vi "Main_v4.vi"() -> ()   [LabVIEW 2016]
uses:
  <vilib>/Analysis/Matrix/Datatypes/RealMatrix.ctl
  subVIs/Global Variables.vi
  <vilib>/picture/3D Picture Control/Helpers/Apply Texture (no reference).vi
  <vilib>/picture/3D Picture Control/NI_3D Picture Control.lvlib
  <vilib>/Analysis/Matrix/NI_Matrix.lvlib
panel:
  in  "Run 2":bool=TRUE
  in  "Refresh Button":bool
  out "Ready?":bool
  in  "Done":bool
  in  "Help":bool
  in  "Abort":bool
  in  "Run":bool
  out "Estimated Time\nfor Lithography":timestamp=timestamp(-68372.87678205769 s since 1904-01-01) format="%<%H:%M:%S>T"
  in  "Visualization":T1(tab)
  out "Render":T2(plugin-control)
  out "Voltage Mapping":dbl(ramp)
  out "2D":T2(plugin-control)
  out "3D Picture":refnum<vi>(3d-picture)
  in  "Settings":T3(tab)
  in  "interpolation distance":dbl=0.1
  in  "Lithography Config File (.lcf)":path=path "P:/users1/Akash/Old/Akash AFM/Test Images/Sample AFM SVGs/2 electrode Writing Test.svg"
  in  "Patterns (drag-and-drop reorder)":i32(listbox)
  in  "image data max":dbl(slide)=100.0 min=0.0 max=100.0 scale=0.0..100.0
  in  "image data min":dbl(slide)=17.365269461077844 min=0.0 max=100.0 scale=0.0..100.0
  in  "AFM Type":u16(ring)=1 items=["Cypher", "MFP3D", "MFP3D_Lucy", "Simulation"]
  in  "Page":i32=1 min=0
  in  "Inkscape File (.svg)":path=path "\\\\synology.phyast.pitt.edu\\public/users1/Yuhe/cypher/1D Coulomb Drag_single QPC.svg"
  in  "Background Image":path=path "\\\\synology.phyast.pitt.edu\\public/users1/Yuhe/AFM scanned images/20170708/SA2821D0001.ibw"
  # "``"
  # "Before you start the program\nchange these paths to the\ncorresponding files"
  # "In simulation mode, to change the perspective, hold the left button of mouse and drag in the picture.\nTo zoom in and out, hold the shift button, hold the left button of the mouse and drag up and down in\nthe picture."
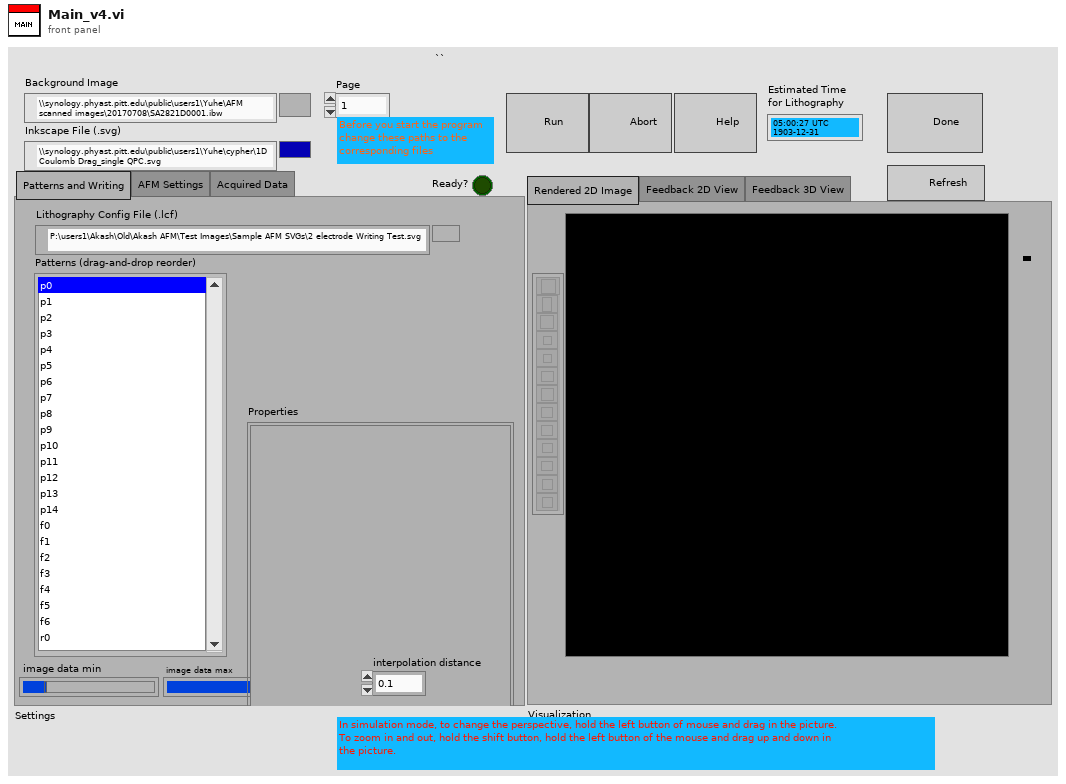
[diagram p1: front panel]
types:
  T1 = enum32{"Rendered 2D Image", "Feedback 2D View", "Feedback 3D View"}
  T2 = typedef "IMAQ Image.ctl" = refnum<image>
  T3 = enum32{"Patterns and Writing", "AFM Settings", "Acquired Data"}
  T4 = enum32{"invalid app kind", "Development System", "Run Time System", "Student Edition", "Embedded LabVIEW", "Evaluation", "Custom"}
  T5 = typedef "NI_Matrix.lvlib/RealMatrix.ctl" = dbl[][]
  T6 = cluster{"paths":cluster{"Fill Color":string, "Stroke Color":string, "Commands":cluster{"Command Type":string, "Coordinates":cluster{"X":dbl, "Y":dbl}[]}[], "Transformation Matrix 2":T5}[], "funnels":cluster{"Fill Color":string, "Stroke Color":string, "Commands":cluster{"Command Type":string, "Coordinates":cluster{"X":dbl, "Y":dbl}[]}[], "Transformation Matrix 2":T5}[], "rects":cluster{"Fill Color":string, "Stroke Color":string, "Width":dbl, "Height":dbl, "X":dbl, "Y":dbl, "Transformation Matrix":T5}[]}
  T7 = cluster{"SceneObject out":refnum<vi>, "Tip":refnum<vi>, "Canvas":refnum<vi>}
  T8 = cluster{"Name":string, "Litho":cluster{"X":dbl, "Y":dbl, "Speed":dbl, "Voltage":dbl}[]}[]
  T9 = cluster{"X":dbl, "Y":dbl, "Speed":dbl, "Voltage":dbl}
  T10 = enum32{"Invalid", "Standard", "Closed", "Hidden", "Minimized", "Maximized"}
  T11 = typedef "Rectangle Properties - cluster.ctl" = cluster{"Enabled":bool, "Direction":u16, "Fill Orientation":u16, "Fill Spacing":dbl, "Speed (um/s)":T12, "Voltage (V)":T12}
  T12 = typedef "Voltage - cluster.ctl" = cluster{"Schedule":T13, "Value":dbl, "Start Value":dbl, "End Value":dbl, "Min Value":dbl, "Max Value":dbl, "Duty Cycle (%)":dbl, "Signal Type":T14, "Cycle Number":dbl, "Phase (degrees)":dbl, "formula":string, "formula length (nm)":dbl, "formula resolution (nm)":dbl}
  T13 = typedef "Schedule - enum.ctl" = enum16{"Constant", "Ramp", "Fn. Generator", "Formula"}
  T14 = typedef "Signal Type - enum.ctl" = enum16{"Sine Wave", "Triangle Wave", "Square Wave", "Sawtooth Wave"}
  T15 = typedef "Funnel Properties - cluster.ctl" = cluster{"Enabled":bool, "Direction":u16, "Smooth Segments":dbl, "Bottom Segs.":dbl, "Speed (um/s)":T12, "Voltage (V)":T12}
  T16 = typedef "Path Properties - cluster.ctl" = cluster{"Enabled":bool, "Direction":u16, "Fill Orientation":u16, "Smooth Segments":dbl, "Fill Spacing":dbl, "Speed (um/s)":T12, "Voltage (V)":T12}
  T17 = cluster{"Path Properties":T16[], "Rectangle Properties":T11[], "Funnel Properties":T15[]}
  T18 = typedef "imagedata.ctl" = cluster{"image type":i32, "image depth":i32, "image":u8[], "mask":u8[], "colors":u32[], "Rectangle":cluster{"left":i16, "top":i16, "right":i16, "bottom":i16}}
  T19 = cluster{"Core":cluster{"Current VI Reference":refnum<vi>, "Close Panel on Exit?":bool}, "Parsing Data":cluster{"paths":cluster{"Fill Color":string, "Stroke Color":string, "Commands":cluster{"Command Type":string, "Coordinates":cluster{"X":dbl, "Y":dbl}[]}[], "Transformation Matrix 2":T5}[], "funnels":cluster{"Fill Color":string, "Stroke Color":string, "Commands":cluster{"Command Type":string, "Coordinates":cluster{"X":dbl, "Y":dbl}[]}[], "Transformation Matrix 2":T5}[], "rects":cluster{"Fill Color":string, "Stroke Color":string, "Width":dbl, "Height":dbl, "X":dbl, "Y":dbl, "Transformation Matrix":T5}[]}, "Lithography Data":cluster{"Name":string, "Litho":cluster{"X":dbl, "Y":dbl, "Speed":dbl, "Voltage":dbl}[]}[], "VI Refs":refnum<vi>[], "Data Queue":refnum<queue>, "3D":cluster{"SceneObject out":refnum<vi>, "Tip":refnum<vi>, "Canvas":refnum<vi>}}
  T20 = cluster{"Current VI Reference":refnum<vi>, "Close Panel on Exit?":bool}
  T21 = cluster{" paths":cluster{"Fill Color":string, "Stroke Color":string, "Commands":cluster{"Command Type":string, "Coordinates":cluster{"X":dbl, "Y":dbl}[]}[], "Transformation Matrix 2":T5}[], " funnels":cluster{"Fill Color":string, "Stroke Color":string, "Commands":cluster{"Command Type":string, "Coordinates":cluster{"X":dbl, "Y":dbl}[]}[], "Transformation Matrix 2":T5}[], "rects":cluster{"Fill":string, "Stroke":string, "width":dbl, "height":dbl, "x":dbl, "y":dbl, "Transformation Matrix":T5}[]}
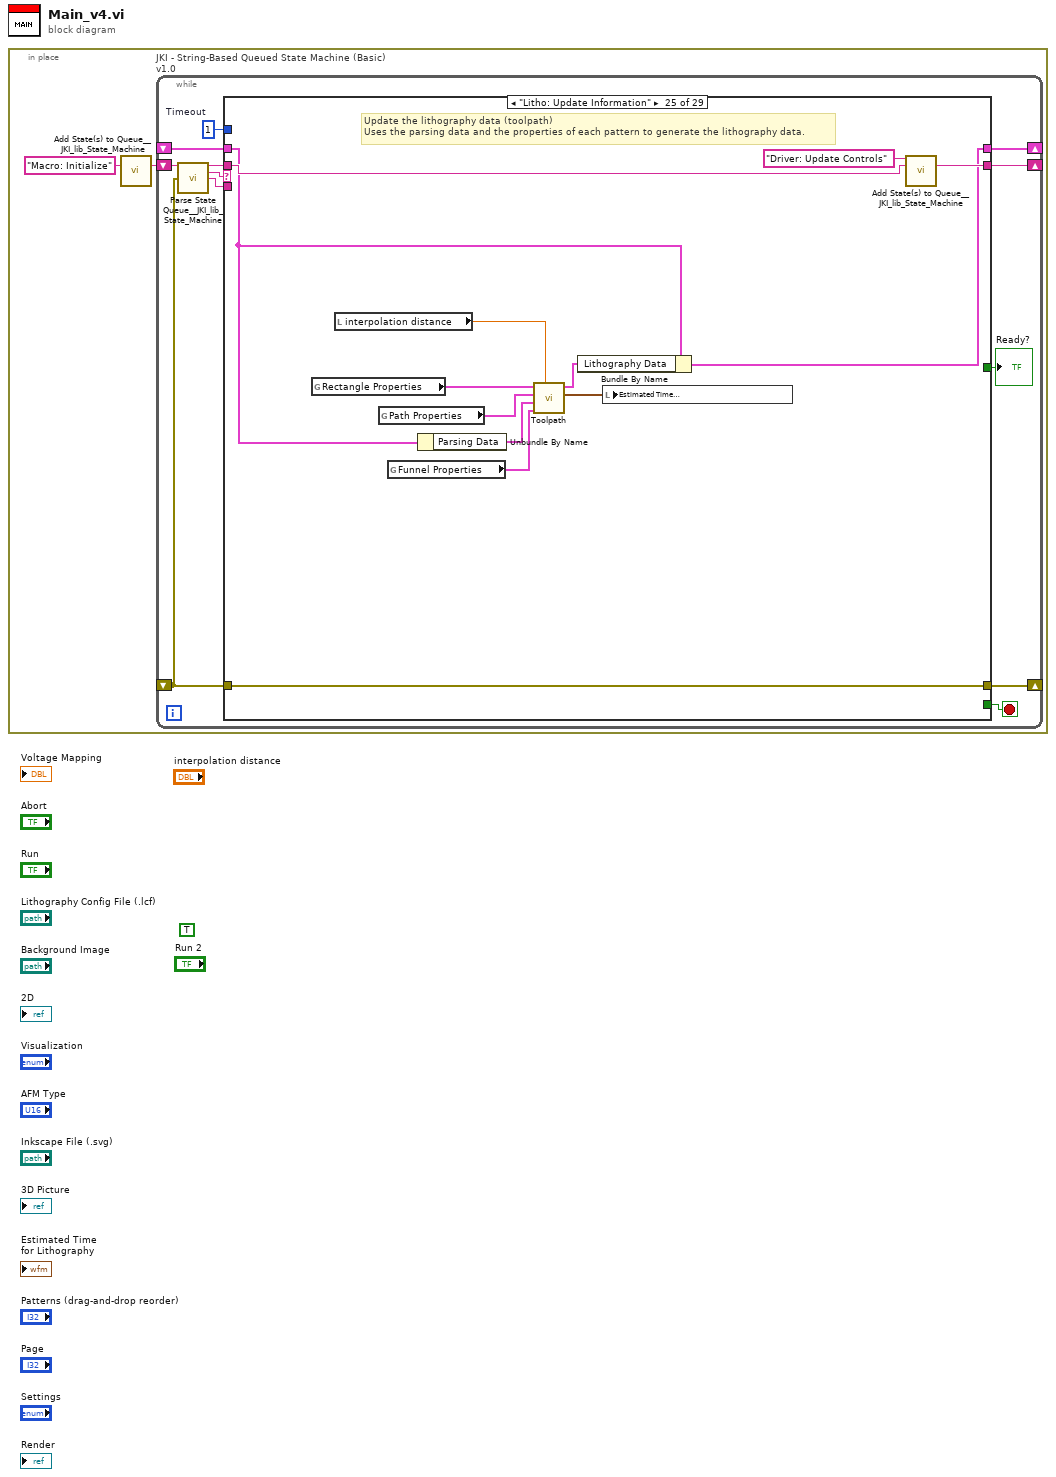
[diagram p0: block diagram]
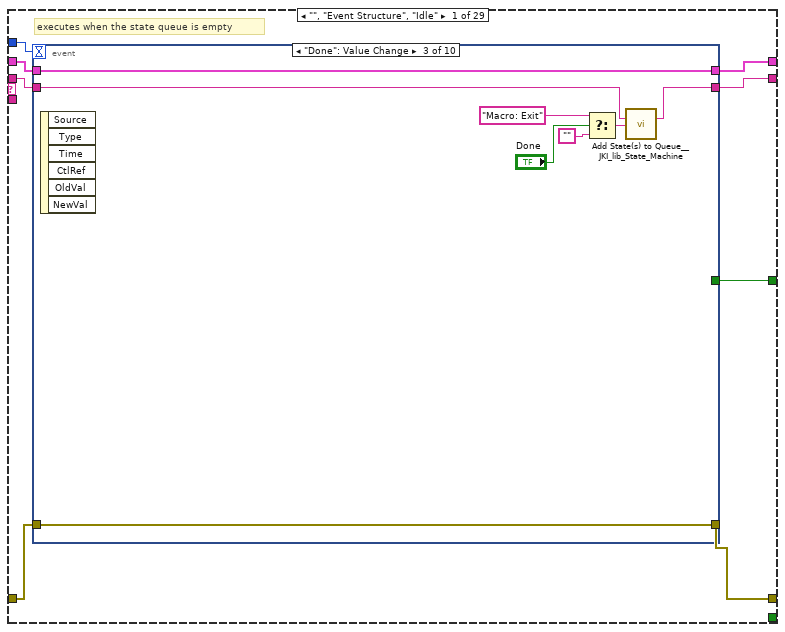
[diagram p2: hidden frame]
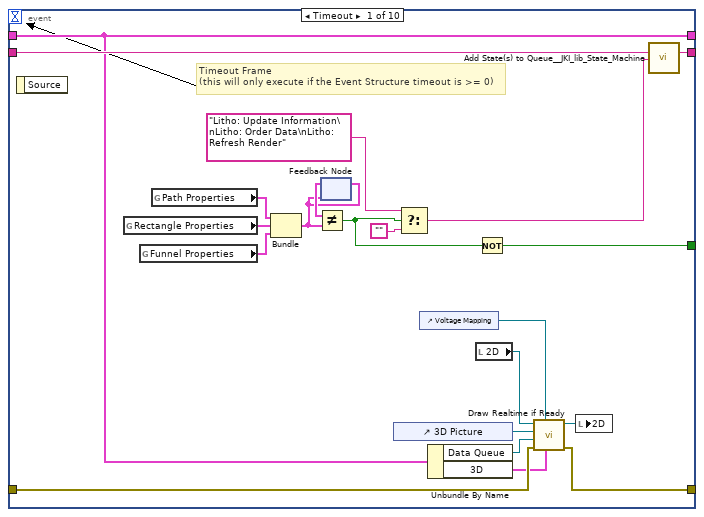
[diagram p3: hidden frame]
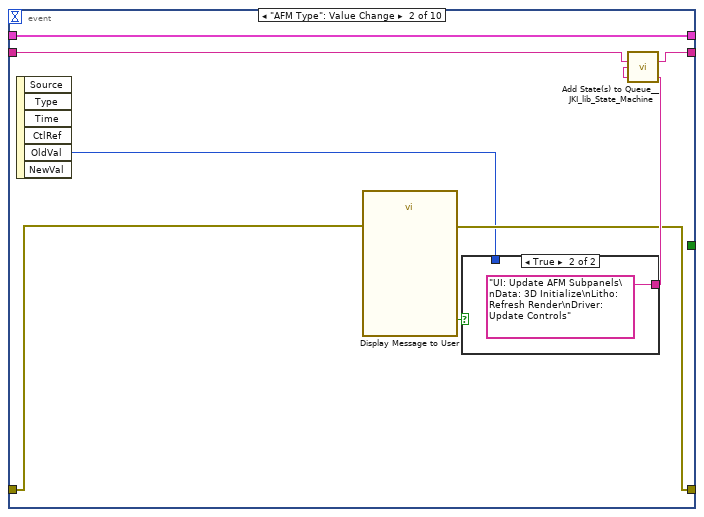
[diagram p4: hidden frame]
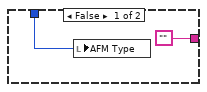
[diagram p5: hidden frame]
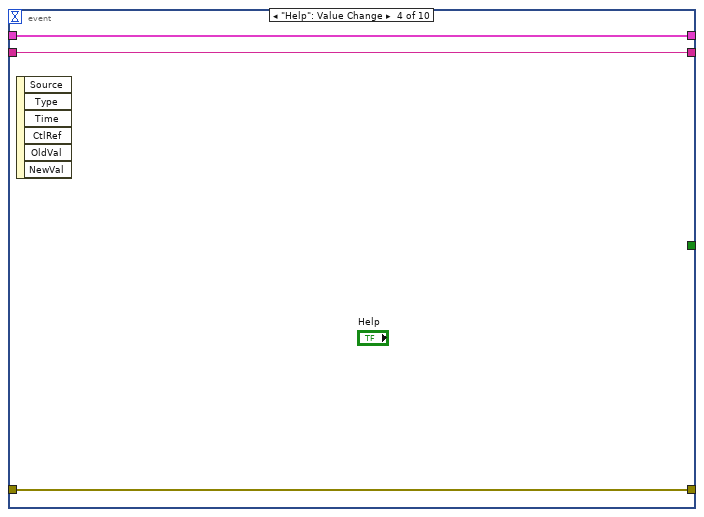
[diagram p6: hidden frame]
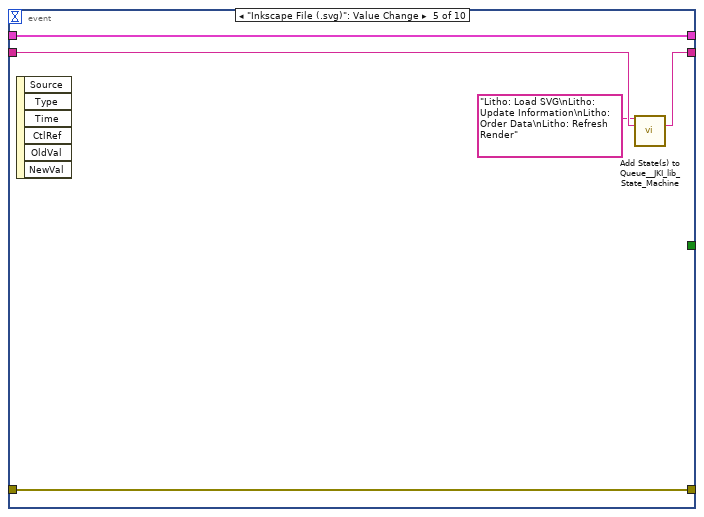
[diagram p7: hidden frame]
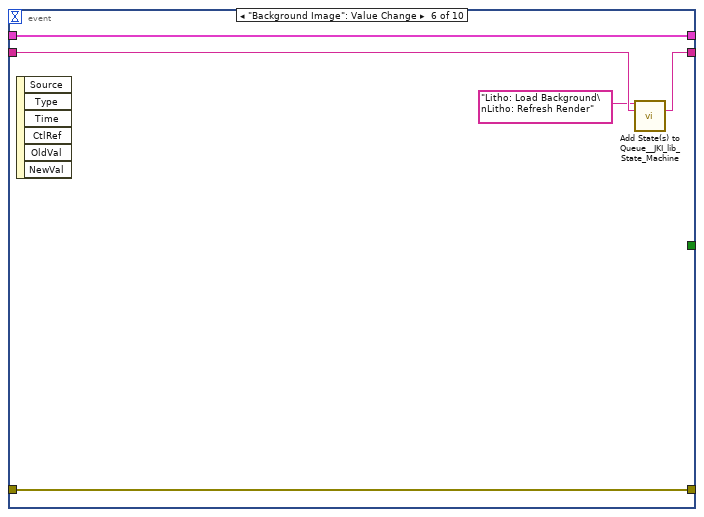
[diagram p8: hidden frame]
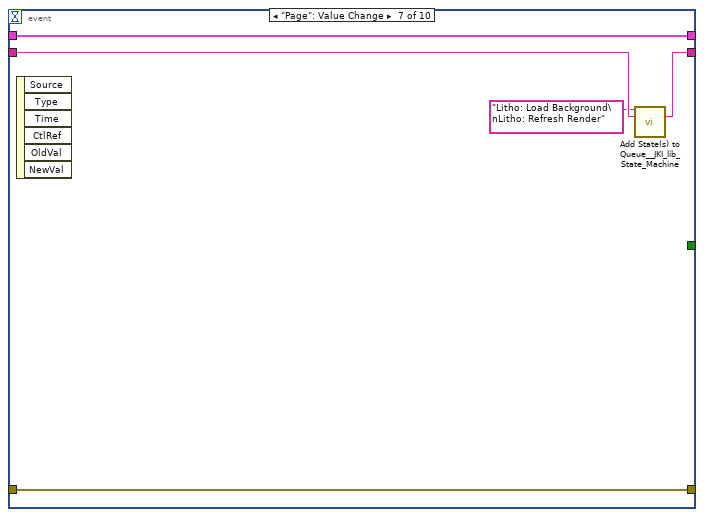
[diagram p9: hidden frame]
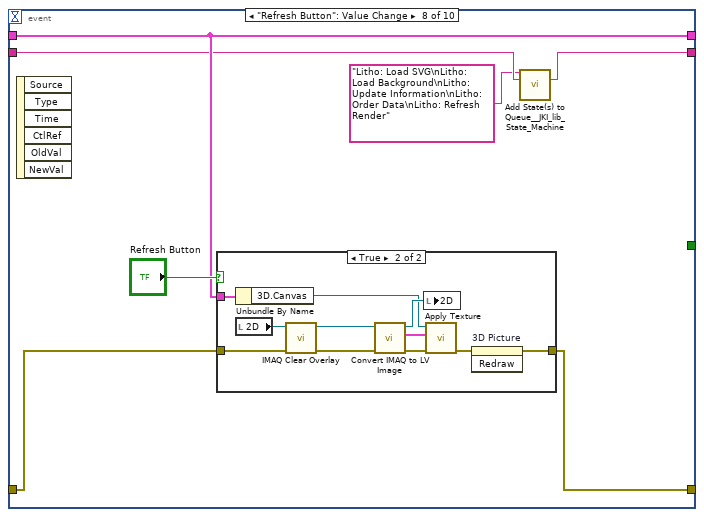
[diagram p10: hidden frame]
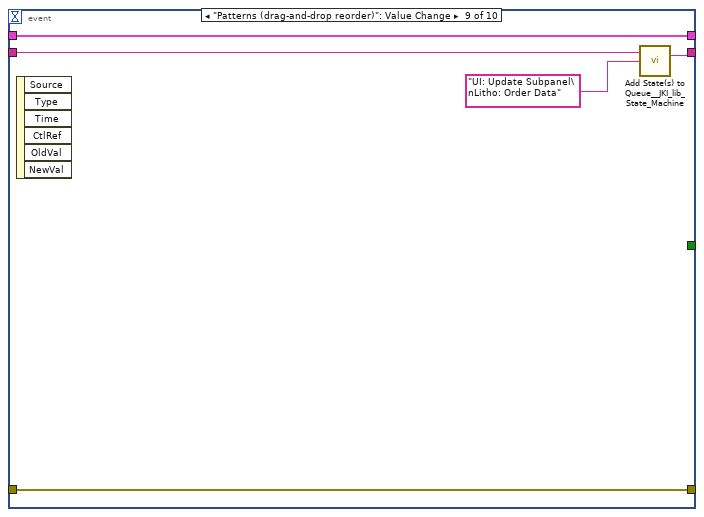
[diagram p12: hidden frame]
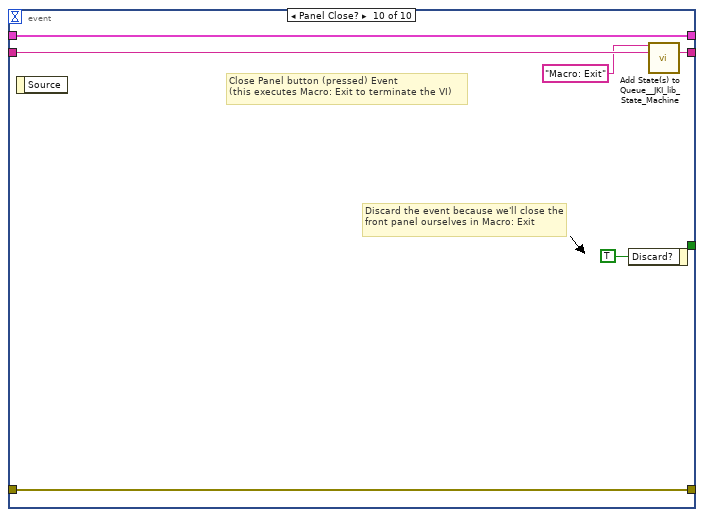
[diagram p13: hidden frame]
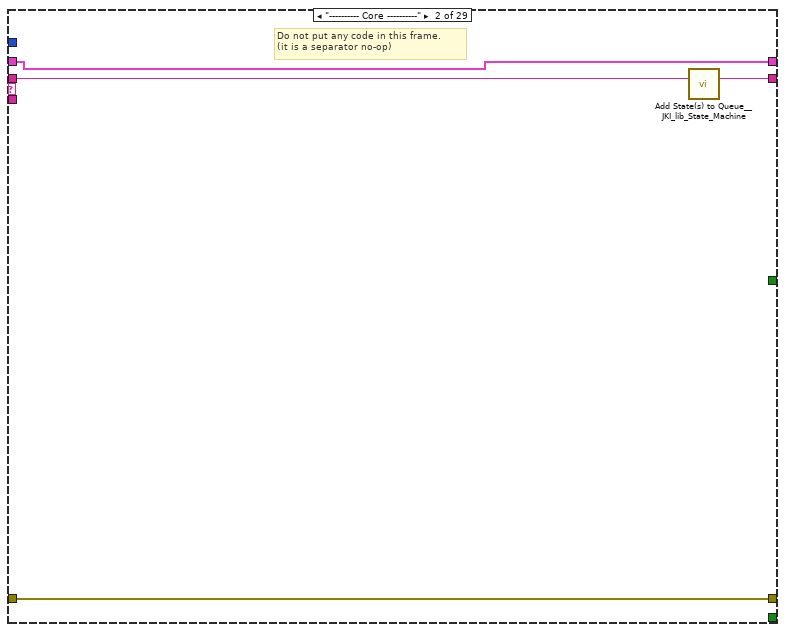
[diagram p14: hidden frame]
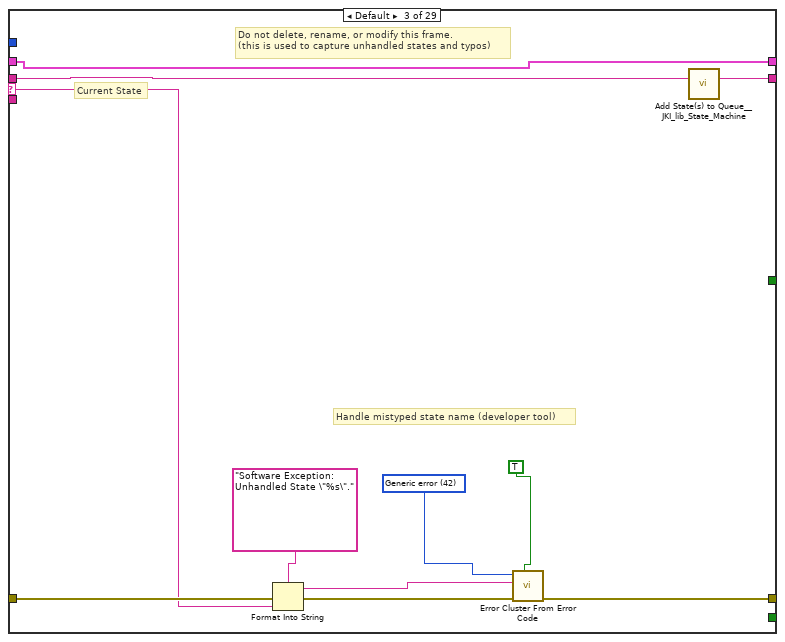
[diagram p15: hidden frame]
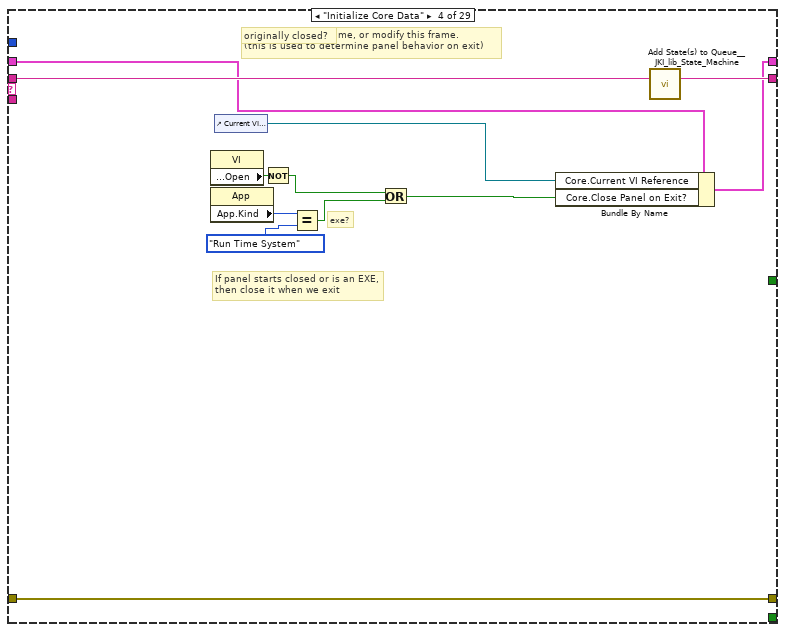
[diagram p16: hidden frame]
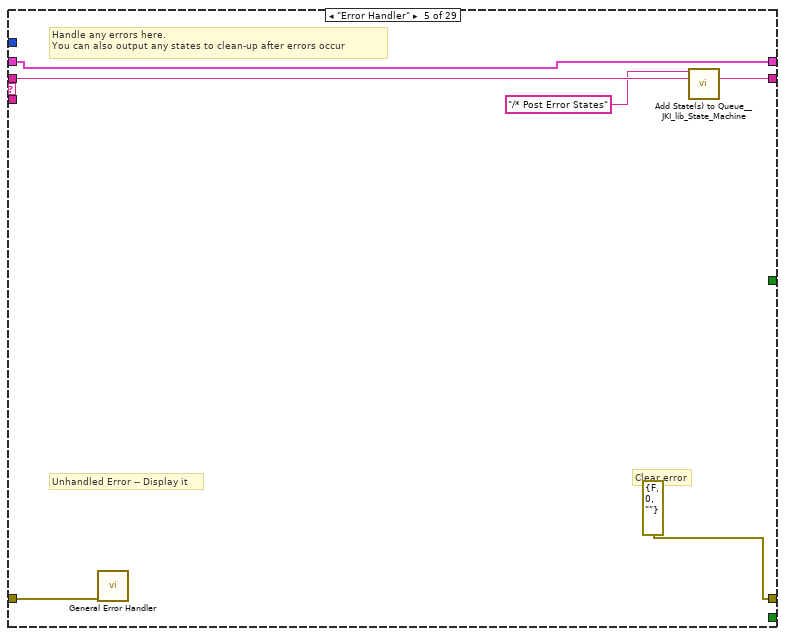
[diagram p17: hidden frame]
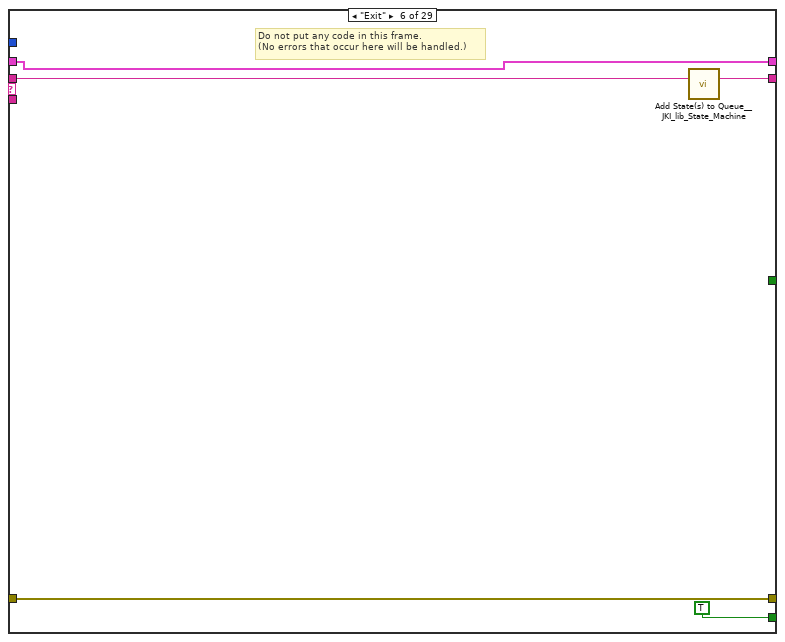
[diagram p18: hidden frame]
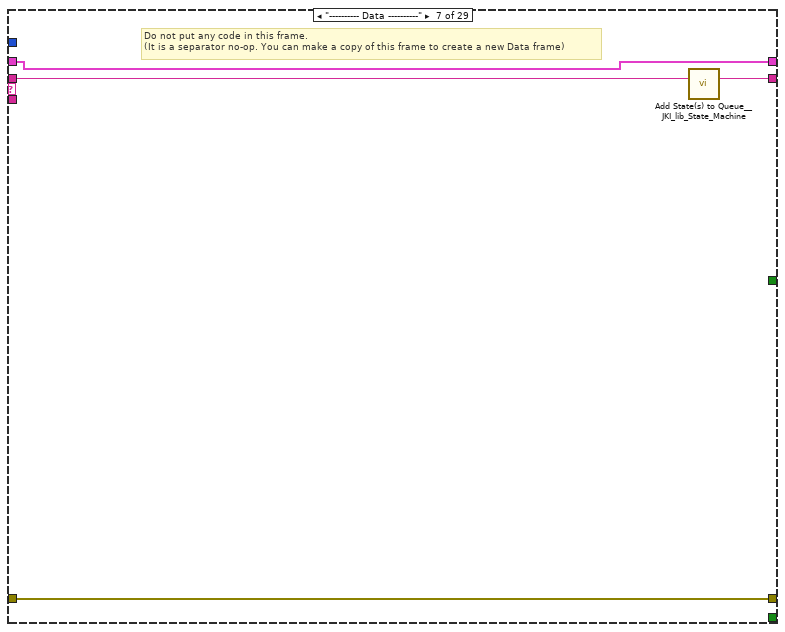
[diagram p19: hidden frame]
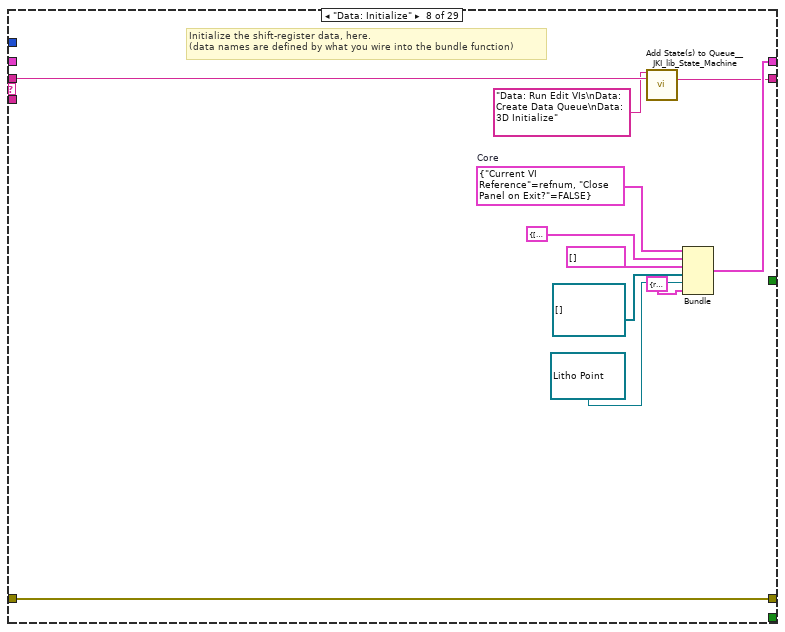
[diagram p20: hidden frame]
diagram:
  (unwired) TRUE
  n1 = in-place {
    n2 = call <vilib>:"Add State(s) to Queue__JKI_lib_State_Machine.vi"("State(s) in (\"\")"="Macro: Initialize") -> ("States Out"=w2:string)  [unwired: 14 in]
    n3 = while "JKI - String-Based Queued State Machine (Basic) v1.0" {
      shift-right: [w7] -> _
      shift-left: _ -> [w6]
      shift-right: [w10] -> _
      shift-left: _ -> [w4]
      shift-right: [w9] -> _
      shift-left: w2 -> [w11]
      stop <- w8 stop-if-true
      w5 = 1  # Timeout
      n4 = call <vilib>:"Parse State Queue__JKI_lib_State_Machine.vi"("State Queue"=w11, "Error In (no error)"=w4) -> ("Remaining States"=w13:string, "Current State"=w14:string, "Arguments"=w12:string)  [unwired: 11 in]
      n5 = case shown="\"Litho: Update Information\"" w14 {
        selector: w14 -> [_ _ w115 _ _ _ _ _ _ _ _ _ _ _ _ _ _ _ _ _ _ _ _ _ _ _ _ _ _]
        tunnel: w13 -> [w22 w114 w119 w137 w143 w148 w152 w158 w166 w183 w202 w220 w227 w240 w256 w274 w280 w291 w317 w322 w332 w336 w345 w360 w373 w383 w398 w402 w417]
        tunnel: w12 -> [_ _ _ _ _ _ _ _ _ _ _ _ _ _ _ _ w275 w285 _ _ _ _ _ _ _ _ _ _ _]
        tunnel: w6 -> [w20 w111 w117 w128 w140 w146 w149 _ w165 w182 w201 w208 w224 w238 w243 w262 w278 w287 w314 w319 w329 w333 w339 w358 w368 w380 w388 w399 w406]
        tunnel: [w19 w112 w121 w134 errorcluster {"status"=FALSE, "code"=0, "source"=""} ("error out") w145 w150 w163 w164 w179 w194 w207 w225 w232 w241 w260 w276 w288 w315 w320 w330 w334 w341 w349 w371 w375 w385 w400 w407] -> w10
        tunnel: w4 -> [w18 w112 w120 w134 w139 w145 w150 w163 w167 w184 w193 w206 w225 w233 w242 w261 w277 w289 w315 w320 w330 w334 w342 w351 w371 w376 w384 w400 w405]
        tunnel: [w21 w113 w118 w136 w142 w147 w151 w156 w166 w183 w202 w219 w226 w239 w255 w273 w279 w290 w316 w321 w331 w335 w344 w359 w372 w382 w397 w401 w416] -> w9
        tunnel: [_ _ _ _ _ TRUE _ _ _ _ _ _ _ _ _ _ _ _ _ _ _ _ _ _ _ _ _ _ _] -> w8
        tunnel: [w17 w111 w117 w135 w140 w146 w149 w157 w168 w185 w203 w208 w224 w238 w243 w262 w278 w287 w314 w319 w329 w333 w338 w358 w367 w379 w388 w399 w406] -> w7
        tunnel: w5 -> [w16 _ _ _ _ _ _ _ _ _ _ _ _ _ _ _ _ _ _ _ _ _ _ _ _ _ _ _ _]
        tunnel: [w15 _ _ _ _ _ _ _ _ _ _ _ _ _ _ _ _ _ _ _ _ _ _ _ _ _ _ _ _] -> w3
        frame "", "Event Structure", "Idle" {
          # "executes when the state queue is empty"
          n6 = event shown="[2] \"Done\": Value Change" {
            selector: _ -> [_ _ _ _ _ _ _ _ _ _]
            dyn-events: _ -> [_ _ _ _ _ _ _ _ _ _]
            timeout: w16 -> [_ _ _ _ _ _ _ _ _ _]
            tunnel: w22 -> [w43 w49 w59 w64 w70 w75 w80 w83 w103 w110]
            tunnel: [w42 w50 w60 w64 w69 w74 w79 w82 w102 w109] -> w21
            tunnel: w20 -> [w26 w51 w62 w65 w67 w72 w77 w84 w104 w107]
            tunnel: [w29 w46 w61 w63 w68 w73 w78 w85 w101 w108] -> w19
            tunnel: w18 -> [w30 w45 w61 w63 w68 w73 w78 w86 w101 w108]
            tunnel: [w26 w51 w62 w65 w67 w72 w77 w84 w104 w107] -> w17
            tunnel: [w24 _ _ _ _ _ _ _ _ _] -> w15
            event Timeout {
              # "Timeout Frame\n(this will only execute if the Event Structure timeout is >= 0)"
              n7 = event-data() -> ()  [unwired: 1 in, 1 out]
              n8 = global read "Global Variables.vi" "Rectangle Properties"() -> (w39:T11[])
              n9 = global read "Global Variables.vi" "Funnel Properties"() -> (w40:T15[])
              n10 = global read "Global Variables.vi" "Path Properties"() -> (w38:T16[])
              n11 = Bundle("Path Properties"=w38, "Rectangle Properties"=w39, "Funnel Properties"=w40) -> (w37:T17)  [unwired: 1 in]
              n12 = feedback #1(w37) -> (w41:T17)
              n13 = Not Equal?(x=w41, y=w37) -> (x != y?=w23:bool)
              n14 = feedback-in #1(w37) -> ()
              n15 = control-ref of="3D Picture"() -> (w32:refnum<vi>)
              n16 = Select(t="Litho: Update Information\nLitho: Order Data\nLitho: Refresh Render", s=w23, f="") -> (s? t:f=w34:string)
              n17 = control-ref of="Voltage Mapping"() -> (w33:refnum<vi>)
              n18 = Unbundle By Name(w26) -> ("Data Queue"=w28:refnum<queue>, "3D"=w27:T7)
              n19 = local read "2D"() -> (w31:T2)
              n20 = Not(x=w23) -> (.not. x?=w24:bool)
              n21 = call "Draw Realtime if Ready.vi"("3D"=w27, "Voltage Mapping"=w33, "error in (no error)"=w30, "Data Queue"=w28, "3D Picture"=w32, "Refnum in"=w31) -> ("error out"=w29:errorcluster, "Image out"=w25:T2)  [unwired: 4 in]
              n22 = local write "2D"(w25) -> ()
              n23 = call <vilib>:"Add State(s) to Queue__JKI_lib_State_Machine.vi"("State(s) in (\"\")"=w43, "State(s) at Back (\"\")"=w34) -> ("States Out"=w42:string)  [unwired: 13 in]
            }
            event "AFM Type": Value Change {
              n24 = event-data() -> ("OldVal"=w44:u16)  [unwired: 1 in, 5 out]
              n25 = call "Display Message to User"("error in (no error)"=w45) -> ("error out"=w46:errorcluster, "OK"=w47:bool)  [unwired: 9 in]
              n26 = case shown="True" w47 {
                tunnel: ["" "UI: Update AFM Subpanels\nData: 3D Initialize\nLitho: Refresh Render\nDriver: Update Controls" ("State(s) at Back (\"\")")] -> w48
                tunnel: w44 -> [w52 _]
                frame False {
                  n27 = local write "AFM Type"(w52) -> ()
                }
                frame True {
                }
              }
              n28 = call <vilib>:"Add State(s) to Queue__JKI_lib_State_Machine.vi"("State(s) in (\"\")"=w49, "State(s) at Back (\"\")"=w48) -> ("States Out"=w50:string)  [unwired: 13 in]
            }
            event "Done": Value Change {
              n29 = event-data() -> ()  [unwired: 1 in, 6 out]
              n30 = Select(t="Macro: Exit", s="Done", f="") -> (s? t:f=w55:string)
              n31 = call <vilib>:"Add State(s) to Queue__JKI_lib_State_Machine.vi"("State(s) in (\"\")"=w59, "State(s) at Back (\"\")"=w55) -> ("States Out"=w60:string)  [unwired: 13 in]
            }
            event "Help": Value Change {
              n32 = event-data() -> ()  [unwired: 1 in, 6 out]
            }
            event "Inkscape File (.svg)": Value Change {
              n33 = event-data() -> ()  [unwired: 1 in, 6 out]
              n34 = call <vilib>:"Add State(s) to Queue__JKI_lib_State_Machine.vi"("State(s) in Front (\"\")"="Litho: Load SVG\nLitho: Update Information\nLitho: Order Data\nLitho: Refresh Render", "State(s) in (\"\")"=w70) -> ("States Out"=w69:string)  [unwired: 13 in]
            }
            event "Background Image": Value Change {
              n35 = event-data() -> ()  [unwired: 1 in, 6 out]
              n36 = call <vilib>:"Add State(s) to Queue__JKI_lib_State_Machine.vi"("State(s) in Front (\"\")"="Litho: Load Background\nLitho: Refresh Render", "State(s) in (\"\")"=w75) -> ("States Out"=w74:string)  [unwired: 13 in]
            }
            event "Page": Value Change {
              n37 = event-data() -> ()  [unwired: 1 in, 6 out]
              n38 = call <vilib>:"Add State(s) to Queue__JKI_lib_State_Machine.vi"("State(s) in Front (\"\")"="Litho: Load Background\nLitho: Refresh Render", "State(s) in (\"\")"=w80) -> ("States Out"=w79:string)  [unwired: 13 in]
            }
            event "Refresh Button": Value Change {
              n39 = event-data() -> ()  [unwired: 1 in, 6 out]
              n40 = case shown="True" "Refresh Button" {
                tunnel: w86 -> [w88 w98]
                tunnel: [w88 w91] -> w85
                tunnel: w84 -> [_ w90]
                frame False {
                }
                frame True {
                  n41 = Unbundle By Name(w90) -> ("3D.Canvas"=w89:refnum<vi>)
                  n42 = local read "2D"() -> (w99:T2)
                  n43 = call "IMAQ Clear Overlay"("error in (no error)"=w98, "Image"=w99) -> ("error out"=w94:errorcluster, "Image Out"=w93:T2)  [unwired: 8 in]
                  n44 = call "Convert IMAQ to LV Image.vi"("error in (no error)"=w94, "IMAQImage In (RGB 32)"=w93) -> ("error out"=w95:errorcluster, "Output Image"=w96:T18, "IMAQImage Out"=w92:T2)  [unwired: 7 in]
                  n45 = local write "2D"(w92) -> ()
                  n46 = call-poly <vilib>:"Apply Texture.vi"("error in (no error)"=w95, "Image Data"=w96, "Scene Object In"=w89) -> ("error out"=w97:errorcluster)  [unwired: 7 in, 1 out]
                  n47 = invoke on="3D Picture" class="SceneGraphDisp (strict)" method="Redraw"(error in=w97) -> (error out=w91:errorcluster)  [unwired: 2 in, 2 out]
                }
              }
              n48 = call <vilib>:"Add State(s) to Queue__JKI_lib_State_Machine.vi"("State(s) in Front (\"\")"="Litho: Load SVG\nLitho: Load Background\nLitho: Update Information\nLitho: Order Data\nLitho: Refresh Render", "State(s) in (\"\")"=w83) -> ("States Out"=w82:string)  [unwired: 13 in]
            }
            event "Patterns (drag-and-drop reorder)": Value Change {
              n49 = event-data() -> ()  [unwired: 1 in, 6 out]
              n50 = call <vilib>:"Add State(s) to Queue__JKI_lib_State_Machine.vi"("State(s) in (\"\")"=w103, "State(s) at Back (\"\")"="UI: Update Subpanel\nLitho: Order Data" ("State(s) at Back (\"\")")) -> ("States Out"=w102:string)  [unwired: 13 in]
            }
            event Panel Close? {
              # "Discard the event because we'll close the front panel ourselves in Macro: Exit"
              # "Close Panel button (pressed) Event\n(this executes Macro: Exit to terminate the VI)"
              n51 = event-data() -> ()  [unwired: 1 in, 1 out]
              n52 = event-data("Discard?"=TRUE) -> ()  [unwired: 1 in, 1 out]
              n53 = call <vilib>:"Add State(s) to Queue__JKI_lib_State_Machine.vi"("State(s) in Front (\"\")"="Macro: Exit", "State(s) in (\"\")"=w110) -> ("States Out"=w109:string)  [unwired: 13 in]
            }
          }
        }
        frame "---------- Core ----------" {
          # "Do not put any code in this frame.\n(it is a separator no-op)"
          n54 = call <vilib>:"Add State(s) to Queue__JKI_lib_State_Machine.vi"("State(s) in (\"\")"=w114) -> ("States Out"=w113:string)  [unwired: 14 in]
        }
        frame Default {
          w124 = 42 items=["No error", "Argument error", "Memory is full", "Out of zone", "End of file", "File already open", "Generic file I/O error", "File not found", "File permission error", "Disk is full", "Duplicate path", "Too many files open", "System feature not enabled", "Resource file not found", "Cannot add resource", "Resource not found", "Image not found", "Image memory error", "Pen does not exist", "Config type invalid", "Config token not found", "Config parse error", "Config memory error", "Bad external code format", "Bad external code offset", "External code not present", "Null window", "Destroy window error", "Null menu", "Print aborted", "Bad print record", "Print driver error", "Windows error during printing", "Memory error during printing", "Print dialog error", "Generic print error", "Invalid device refnum", "Device not found", "Device parameter error", "Device unit error", "Cannot open device", "Device call aborted", "Generic error", "Cancelled by user", "Object ID too low", "Object ID too high", "Object not in heap", "Unknown heap", "Unknown object (invalid DefProc)", "Unknown object (DefProc not in table)", "Message out of range", "Invalid (null) method", "Unknown message", "Manager call not supported", "Bad address", "Network operation in progress", "Network operation timed out", "Connection is busy", "Network attribute not supported", "Network error", "Address in use", "System out of memory", "Connection aborted", "Connection refused", "Not connected", "Already connected", "Connection closed", "Initialization error (interapplication manager)", "Bad occurrence", "Wait on unbound occurrence handler", "Occurrence queue overflow", "Datalog type conflict", "Unused", "Unrecognized type (interapplication manager)", "Memory corrupt", "Failed to make temporary DLL", "Old CIN version", "Drag socket not found", "Failed to load drop-object", "Failed to register OLE object", "Failed to release OLE object", "Format specifier type mismatch", "Unknown format specifier", "Too few format specifiers", "Too many format specifiers", "Scan failed", "Newer CIN version", "Error converting to variant", "Runtime menu error", "Password tampered", "Variant attribute not found", "Incompatible variant data type", "Event data is not available", "Event Store is not present", "Occurrence is not found", "Event Queue is not created", "Event info is not available", "Refnum passed is NULL", "Error retrieving Class GUID", "Error retrieving CoClass GUID", "Error retrieving TypeLib GUID.", "Bad built application magic bytes.", "Specific driver is different from the specific driver associated with the Logical Name.", "There is no session opened to the class driver.", "Max Error", "MAX - Error with config objects", "MAX - Error loading configuration", "MAX - Group not supported"]
          # "Current State"
          # "Do not delete, rename, or modify this frame.\n(this is used to capture unhandled states and typos)"
          # "Handle mistyped state name (developer tool)"
          n55 = Format Into String(format string="Software Exception: Unhandled State \"%s\"." ("message"), error in=w120, w115) -> (resulting string=w123:string, error out=w122:errorcluster)  [unwired: 1 in]
          n56 = call <vilib>:"Error Cluster From Error Code.vi"("show call chain? (False)"=TRUE, "error in (no error)"=w122, "error message (\"\")"=w123, "error code (0)"=w124) -> ("error out"=w121:errorcluster)  [unwired: 5 in]
          n57 = call <vilib>:"Add State(s) to Queue__JKI_lib_State_Machine.vi"("State(s) in (\"\")"=w119) -> ("States Out"=w118:string)  [unwired: 14 in]
        }
        frame "Initialize Core Data" {
          # "Do not delete, rename, or modify this frame.\n(this is used to determine panel behavior on exit)"
          # "originally closed?"
          # "exe?"
          # "If panel starts closed or is an EXE, then close it when we exit"
          n58 = property class="VI"() -> ("Front Panel.Open"=w133:bool)  [unwired: 2 in, 2 out]
          n59 = property class="App"() -> ("App.Kind"=w132:T4)  [unwired: 2 in, 2 out]
          n60 = control-ref of="Current VI Reference"() -> (w126:refnum<vi>)
          n61 = Not(x=w133) -> (.not. x?=w130:bool)
          n62 = Equal?(x=w132, y=T4."Run Time System" ("Application:Kind")) -> (x = y?=w129:bool)
          n63 = Or(x=w130, y=w129) -> (x .or. y?=w127:bool)
          n64 = Bundle By Name(cluster=w128, "Core.Current VI Reference"=w126, "Core.Close Panel on Exit?"=w127) -> (w135:T19)
          n65 = call <vilib>:"Add State(s) to Queue__JKI_lib_State_Machine.vi"("State(s) in (\"\")"=w137) -> ("States Out"=w136:string)  [unwired: 14 in]
        }
        frame "Error Handler" {
          # "Unhandled Error -- Display it"
          # "Handle any errors here.\nYou can also output any states to clean-up after errors occur"
          # "Clear error"
          n66 = call <vilib>:"General Error Handler.vi"("error in (no error)"=w139) -> ()  [unwired: 10 in, 5 out]
          n67 = call <vilib>:"Add State(s) to Queue__JKI_lib_State_Machine.vi"("State(s) in Front (\"\")"="/* Post Error States", "State(s) in (\"\")"=w143) -> ("States Out"=w142:string)  [unwired: 13 in]
        }
        frame "Exit" {
          # "Do not put any code in this frame.\n(No errors that occur here will be handled.)"
          n68 = call <vilib>:"Add State(s) to Queue__JKI_lib_State_Machine.vi"("State(s) in (\"\")"=w148) -> ("States Out"=w147:string)  [unwired: 14 in]
        }
        frame "---------- Data ----------" {
          # "Do not put any code in this frame.\n(It is a separator no-op. You can make a copy of this frame to create a new Data frame)"
          n69 = call <vilib>:"Add State(s) to Queue__JKI_lib_State_Machine.vi"("State(s) in (\"\")"=w152) -> ("States Out"=w151:string)  [unwired: 14 in]
        }
        frame "Data: Initialize" {
          w162 = T20 {"Current VI Reference"=refnum, "Close Panel on Exit?"=FALSE}  # Core
          # "Initialize the shift-register data, here.\n(data names are defined by what you wire into the bundle function)"
          n70 = call <vilib>:"Add State(s) to Queue__JKI_lib_State_Machine.vi"("State(s) in Front (\"\")"="Data: Run Edit VIs\nData: Create Data Queue\nData: 3D Initialize" ("State(s) at Back (\"\")"), "State(s) in (\"\")"=w158) -> ("States Out"=w156:string)  [unwired: 13 in]
          n71 = Bundle("Core"=w162, "Parsing Data"=T6 {"paths"=[], "funnels"=[], "rects"=[]}, "Lithography Data"=T8 [], "VI Refs"=refnum<vi>[] [], "Data Queue"=refnum<queue> refnum, "3D"=T7 {"SceneObject out"=refnum, "Tip"=refnum, "Canvas"=refnum}) -> (w157:T19)  [unwired: 1 in]
        }
        frame "Data: Run Edit VIs" {
          w169 = path[] [path "subVIs/subpanel/Path Edit.vi", path "subVIs/subpanel/Rect Edit.vi", path "subVIs/subpanel/Funnel Edit.vi"]  # Edit VIs
          n72 = for {
            tunnel: [w174] -> w170 mode=indexing
            shift-right: [w172] -> w164
            shift-left: w167 -> [w173]
            tunnel: w169 -> [w171] mode=indexing
            # "Load and run Plugin VIs"
            n73 = Open VI Reference(vi path=w171, error in (no error)=w173) -> (vi reference=w175:refnum<vi>, error out=w176:errorcluster)  [unwired: 4 in]
            n74 = invoke class="VI" method="Run VI"(reference=w175, error in=w176, "Wait until done"=FALSE ("Wait Until Done")) -> (reference out=w174:refnum<vi>, error out=w172:errorcluster)  [unwired: 2 in, 3 out]
          }
          n75 = Bundle By Name(cluster=w165, "VI Refs"=w170) -> (w168:T19)
        }
        frame "Data: Create Data Queue" {
          n76 = Obtain Queue(name (unnamed)="Litho Data", element data type=T9 {"X"=0.0, "Y"=0.0, "Speed"=0.0, "Voltage"=0.0} ("Litho Point"), error in (no error)=w184) -> (queue out=w181:refnum<queue>, error out=w180:errorcluster)  [unwired: 2 in, 1 out]
          n77 = Flush Queue(queue=w181, error in (no error)=w180) -> (queue out=w178:refnum<queue>, error out=w179:errorcluster)  [unwired: 1 out]
          n78 = Bundle By Name(cluster=w182, "Data Queue"=w178) -> (w185:T19)
        }
        frame "Data: 3D Initialize" {
          n79 = property on="AFM Type" class="Ring (strict)"() -> ("RingText.Text"=w199:string)  [unwired: 2 in, 2 out]
          n80 = call <vilib>:"Application Directory.vi"() -> ("Application Directory"=w188:path)
          n81 = Build Path(base path=w188, name or relative path=path "AFMs" ("path")) -> (appended path=w189:path)
          n82 = Build Path(base path=w189, name or relative path=w199) -> (appended path=w197:path)
          n83 = Build Path(base path=w197, name or relative path="Tip.wrl") -> (appended path=w200:path)
          n84 = call "Generate 3D Picture.vi"("Tip Model File (.wrl)"=w200, "error in (no error)"=w193) -> ("error out"=w194:errorcluster, "Canvas"=w196:refnum<vi>, "Tip"=w195:refnum<vi>, "SceneObject out"=w191:refnum<vi>)  [unwired: 6 in]
          n85 = local write "3D Picture"(w191) -> ()
          n86 = Bundle("SceneObject out"=w191, "Tip"=w195, "Canvas"=w196) -> (w192:T7)  [unwired: 1 in]
          n87 = Bundle By Name(cluster=w201, "3D"=w192) -> (w203:T19)
        }
        frame "Data: Cleanup" {
          # "Cleanup any data and references, here.\n(this is called automatically, by the Macro: Exit)"
          n88 = property on="Acquired Data" class="SubPnl"() -> ("InsertedVI"=w213:refnum<vi>)  [unwired: 2 in, 2 out]
          n89 = call "Abort If Not Refnum.vi"("error in (no error)"=w206, "VI in"=w213) -> ("error out"=w210:errorcluster)  [unwired: 9 in]
          n90 = invoke on="Acquired Data" class="SubPnl" method="Remove VI"(error in=w210) -> (error out=w209:errorcluster)  [unwired: 2 in, 2 out]
          n91 = property on="AFM Settings" class="SubPnl"() -> ("InsertedVI"=w212:refnum<vi>)  [unwired: 2 in, 2 out]
          n92 = Unbundle By Name(w208) -> ("Core.Current VI Reference"=w217:refnum<vi>, "VI Refs"=w218:refnum<vi>[], "Data Queue"=w216:refnum<queue>)
          n93 = call "Abort If Not Refnum.vi"("error in (no error)"=w209, "VI in"=w212) -> ("error out"=w211:errorcluster)  [unwired: 9 in]
          n94 = invoke on="AFM Settings" class="SubPnl" method="Remove VI"(error in=w211) -> (error out=w205:errorcluster)  [unwired: 2 in, 2 out]
          n95 = for {
            tunnel: w218 -> [w223] mode=indexing
            shift-right: [w221] -> w215
            shift-left: w205 -> [w222]
            n96 = call "Abort If Not Refnum.vi"("error in (no error)"=w222, "VI in"=w223) -> ("error out"=w221:errorcluster)  [unwired: 9 in]
          }
          n97 = Release Queue(queue=w216, force destroy? (F)=TRUE, error in (no error)=w215) -> (error out=w214:errorcluster)  [unwired: 2 out]
          n98 = call <vilib>:"Add State(s) to Queue__JKI_lib_State_Machine.vi"("State(s) in (\"\")"=w220) -> ("States Out"=w219:string)  [unwired: 14 in]
          n99 = Close Reference(reference=w217, error in (no error)=w214) -> (error out=w207:errorcluster)
        }
        frame "---------- UI ----------" {
          # "Do not put any code in this frame.\n(It is a separator no-op. You can make a copy of this frame to create a new UI frame)"
          n100 = call <vilib>:"Add State(s) to Queue__JKI_lib_State_Machine.vi"("State(s) in (\"\")"=w227) -> ("States Out"=w226:string)  [unwired: 14 in]
        }
        frame "UI: Initialize" {
          # "FIX THIS TO IGNORE .svn"
          # "Initialize the User Interface, here.\n(this is called automatically, by the Macro: Init)"
          n101 = call <vilib>:"Application Directory.vi"() -> ("Application Directory"=w235:path)
          n102 = Build Path(base path=w235, name or relative path=path "AFMs" ("path")) -> (appended path=w236:path)
          n103 = List Folder(path=w236, error in=w233) -> (folder names=w230:string[], error out=w234:errorcluster)  [unwired: 2 in, 2 out]
          n104 = Array Subset(array=w230, index=0) -> (w229:string[])  [unwired: 1 in]
          n105 = property on="AFM Type" class="Ring (strict)"(error in=w234, "Strings []"=w229) -> (error out=w232:errorcluster)  [unwired: 1 in, 1 out]
          n106 = call <vilib>:"Add State(s) to Queue__JKI_lib_State_Machine.vi"("State(s) in Front (\"\")"="UI: Update Subpanel\nUI: Update AFM Subpanels" ("State(s) at Back (\"\")"), "State(s) in (\"\")"=w240) -> ("States Out"=w239:string)  [unwired: 13 in]
        }
        frame "UI: Update Subpanel" {
          # "Subpanel is updated to reflect pattern's type."
          n107 = control-ref of="Patterns (drag-and-drop reorder)"() -> (w254:refnum<vi>)
          n108 = call "Get Selected Pattern.vi"("error in (no error)"=w242, "ListBox in"=w254) -> ("error out"=w247:errorcluster, "Pattern Index"=w245:i32, "Type"=w252:string)  [unwired: 7 in]
          n109 = case shown="\"p\"" w252 {
            tunnel: [2 0 1] -> w251
            frame "f", Default {
            }
            frame "p" {
            }
            frame "r" {
            }
          }
          n110 = Unbundle By Name(w243) -> ("VI Refs"=w244:refnum<vi>[])
          n111 = Index Array(array=w244, index=w251) -> (element=w250:refnum<vi>)
          n112 = invoke class="VI" method="Ctrl Val.Set"(reference=w250, error in=w247, "Control Name"="Index", "Value"=w245) -> (reference out=w249:refnum<vi>, error out=w248:errorcluster)  [unwired: 1 in, 3 out]
          n113 = invoke on="Properties" class="SubPanel" method="Remove VI"(error in=w248) -> (error out=w253:errorcluster)  [unwired: 2 in, 2 out]
          n114 = invoke on="Properties" class="SubPanel" method="Insert VI"(error in=w253, "VI Ref"=w249) -> (error out=w241:errorcluster)  [unwired: 2 in, 3 out]
          n115 = call <vilib>:"Add State(s) to Queue__JKI_lib_State_Machine.vi"("State(s) in (\"\")"=w256) -> ("States Out"=w255:string)  [unwired: 14 in]
        }
        frame "UI: Update AFM Subpanels" {
          # "Subpanels are updated to reflect AFM type."
          n116 = control-ref of="Background Image"() -> (w268:refnum<vi>)
          n117 = control-ref of="Inkscape File (.svg)"() -> (w266:refnum<vi>)
          n118 = control-ref of="AFM Settings"() -> (w271:refnum<vi>)
          n119 = control-ref of="Run"() -> (w265:refnum<vi>)
          n120 = control-ref of="Abort"() -> (w264:refnum<vi>)
          n121 = control-ref of="AFM Type"() -> (w267:refnum<vi>)
          n122 = control-ref of="Acquired Data"() -> (w263:refnum<vi>)
          n123 = call "Load AFM Subpanel.vi"("Ring in"=w267, "Background Image"=w268, "name or relative path"="Driver.vi", "Inkscape File (.svg)"=w266, "input cluster"=w262, "Subpanel"=w271, "error in (no error)"=w261, "Run"=w265, "Abort"=w264) -> ("error out"=w270:errorcluster)  [unwired: 5 in, 1 out]
          n124 = call "Load AFM Subpanel.vi"("Ring in"=w267, "Background Image"=w268, "name or relative path"="Acquired Data.vi", "Inkscape File (.svg)"=w266, "input cluster"=w262, "Subpanel"=w263, "error in (no error)"=w270, "Run"=w265, "Abort"=w264) -> ("error out"=w260:errorcluster)  [unwired: 5 in, 1 out]
          n125 = call <vilib>:"Add State(s) to Queue__JKI_lib_State_Machine.vi"("State(s) in (\"\")"=w274) -> ("States Out"=w273:string)  [unwired: 14 in]
        }
        frame "UI: Cursor Set" {
          # "Argument"
          # "Set and Unset Cursor Busy.\n(Usage: \"UI: Cursor Set >> Busy|Idle\")"
          n126 = case shown="\"Idle\", Default" w275 {
            tunnel: w277 -> [w282 w284]
            tunnel: [w281 w283] -> w276
            frame "Idle", Default {
              n127 = call <vilib>:"Unset Busy.vi"("error in (no error)"=w282) -> ("error out"=w281:errorcluster)  [unwired: 10 in]
            }
            frame "Busy" {
              n128 = call <vilib>:"Set Busy.vi"("error in (no error)"=w284) -> ("error out"=w283:errorcluster)  [unwired: 9 in, 1 out]
            }
          }
          n129 = call <vilib>:"Add State(s) to Queue__JKI_lib_State_Machine.vi"("State(s) in (\"\")"=w280) -> ("States Out"=w279:string)  [unwired: 14 in]
        }
        frame "UI: Front Panel State" {
          # "Argument"
          # "Set Front Panel Open or Closed\n(Usage: \"UI: Front Panel State >> Open|Close\")"
          n130 = Unbundle By Name(w287) -> ("Core.Current VI Reference"=w286:refnum<vi>)
          n131 = case shown="\"Open\", Default" w285 {
            tunnel: w289 -> [w295 w308]
            tunnel: [w297 w309] -> w288
            tunnel: w286 -> [w296 w306]
            frame "Open", Default {
              n132 = property class="VI"(reference=w296, error in=w295) -> (reference out=w293:refnum<vi>, error out=w294:errorcluster, "Front Panel.Open"=w292:bool)
              n133 = case shown="True" w292 {
                tunnel: [w300 w303] -> w297
                tunnel: w294 -> [w299 w303]
                tunnel: w293 -> [w298 _]
                frame False {
                  n134 = invoke class="VI" method="FP.Open"(reference=w298, error in=w299, "Activate"=TRUE, "State"=T10."Standard") -> (error out=w300:errorcluster)  [unwired: 1 in, 4 out]
                }
                frame True {
                }
              }
            }
            frame "Close" {
              n135 = property class="VI"(reference=w306, error in=w308) -> (reference out=w305:refnum<vi>, error out=w307:errorcluster, "Front Panel.Open"=w304:bool)
              n136 = case shown="False" w304 {
                tunnel: [w310 w313] -> w309
                tunnel: w307 -> [w310 w312]
                tunnel: w305 -> [_ w311]
                frame False {
                }
                frame True {
                  n137 = invoke class="VI" method="FP.Close"(reference=w311, error in=w312) -> (error out=w313:errorcluster)  [unwired: 1 in, 2 out]
                }
              }
            }
          }
          n138 = call <vilib>:"Add State(s) to Queue__JKI_lib_State_Machine.vi"("State(s) in (\"\")"=w291) -> ("States Out"=w290:string)  [unwired: 14 in]
        }
        frame "---------- Macro ----------" {
          # "Do not put any code in this frame.\n(It is a separator no-op. You can make a copy of this frame to create a new Macro frame)"
          n139 = call <vilib>:"Add State(s) to Queue__JKI_lib_State_Machine.vi"("State(s) in (\"\")"=w317) -> ("States Out"=w316:string)  [unwired: 14 in]
        }
        frame "Macro: Initialize" {
          w318 = "Data: Initialize\nInitialize Core Data\nUI: Initialize\nUI: Front Panel State >> Open\nLitho: Load SVG\nLitho: Load Background\nLitho: Update Information\nLitho: Order Data\nLitho: Refresh Render"  # Data: Initialize Initialize Core Data UI: Initialize UI: Front Panel State >> Open Litho: Load SVG Litho: Load Background Litho: Update Information Litho: Order Data Litho: Refresh Render
          # "Initialization Macro\n(This is called once, when the VI starts)"
          n140 = call <vilib>:"Add State(s) to Queue__JKI_lib_State_Machine.vi"("State(s) in Front (\"\")"=w318, "State(s) in (\"\")"=w322) -> ("States Out"=w321:string)  [unwired: 13 in]
        }
        frame "Macro: Exit" {
          # "Exit Macro\n(This is called once, when the VI exits)"
          n141 = Unbundle By Name(w329) -> ("Core.Close Panel on Exit?"=w328:bool)
          n142 = Select(t="UI: Front Panel State >> Close", s=w328, f="") -> (s? t:f=w325:string)
          n143 = call <vilib>:"Add State(s) to Queue__JKI_lib_State_Machine.vi"("State(s) in (\"\")"=w325, "State(s) at Back (\"\")"="Data: Cleanup\nExit") -> ("States Out"=w323:string)  [unwired: 13 in]
          n144 = call <vilib>:"Add State(s) to Queue__JKI_lib_State_Machine.vi"("State(s) in Front (\"\")"=w323, "State(s) in (\"\")"=w332) -> ("States Out"=w331:string)  [unwired: 13 in]
        }
        frame "---------- Litho ----------" {
          # "Template Separator\n(You can make a copy of, or modify, this frame)"
          n145 = call <vilib>:"Add State(s) to Queue__JKI_lib_State_Machine.vi"("State(s) in (\"\")"=w336) -> ("States Out"=w335:string)  [unwired: 14 in]
        }
        frame "Litho: Load SVG" {
          # "Load SVG\nParses the SVG and stores the data obtained from it."
          n146 = local read "Inkscape File (.svg)"() -> (w343:path)
          n147 = call "SVG Parser.vi"("error in (no error)"=w342, "XML File Path"=w343) -> ("error out"=w341:errorcluster, "Parsing Data"=w340:T21, "Image Size"=w337:cluster{"Width":dbl, "Height":dbl})  [unwired: 1 in]
          n148 = global write "Global Variables.vi" "Size"(w337) -> ()
          n149 = Bundle By Name(cluster=w339, "Parsing Data"=w340) -> (w338:T19)
          n150 = call <vilib>:"Add State(s) to Queue__JKI_lib_State_Machine.vi"("State(s) in (\"\")"=w345) -> ("States Out"=w344:string)  [unwired: 14 in]
        }
        frame "Litho: Load Background" {
          # "Load Background\nLoads the background file into the images."
          n151 = local read "Background Image"() -> (w352:path)
          n152 = local read "Page"() -> (w353:i32)
          n153 = call "Background.vi"("image data max"="image data max", "image data min"="image data min", "error in (no error)"=w351, "Page"=w353, "Image File Path"=w352) -> ("error out"=w356:errorcluster, "Background out"=w348:T2)  [unwired: 5 in]
          n154 = local write "Render"(w348) -> ()
          n155 = call "Imaq Create"("Image Name"="2D", "error in (no error)"=w356) -> ("New Image"=w357:T2, "error out"=w354:errorcluster)  [unwired: 3 in]
          n156 = call "IMAQ Copy"("error in (no error)"=w354, "Image Dst"=w357, "Image Src"=w348) -> ("error out"=w349:errorcluster, "Image Dst Out"=w350:T2)  [unwired: 3 in]
          n157 = local write "2D"(w350) -> ()
          n158 = call <vilib>:"Add State(s) to Queue__JKI_lib_State_Machine.vi"("State(s) in (\"\")"=w360) -> ("States Out"=w359:string)  [unwired: 14 in]
        }
        frame "Litho: Update Information" {
          # "Update the lithography data (toolpath)\nUses the parsing data and the properties of each pattern to generate the lithography data."
          n159 = global read "Global Variables.vi" "Rectangle Properties"() -> (w366:T11[])
          n160 = local read "interpolation distance"() -> (w361:dbl)
          n161 = global read "Global Variables.vi" "Path Properties"() -> (w365:T16[])
          n162 = global read "Global Variables.vi" "Funnel Properties"() -> (w364:T15[])
          n163 = Unbundle By Name(w368) -> ("Parsing Data"=w370:T6)
          n164 = call "Toolpath.vi"("interpolation distance"=w361, "Funnel Properties"=w364, "Parsing Data"=w370, "Path Properties"=w365, "Rectangle Properties"=w366) -> ("Estimated Time Required"=w363:timestamp, "Lithography Data"=w369:T8)  [unwired: 3 in]
          n165 = Bundle By Name(cluster=w368, "Lithography Data"=w369) -> (w367:T19)
          n166 = local write "Estimated Time\nfor Lithography"(w363) -> ()
          n167 = call <vilib>:"Add State(s) to Queue__JKI_lib_State_Machine.vi"("State(s) in Front (\"\")"="Driver: Update Controls" ("State(s) in Front (\"\")"), "State(s) in (\"\")"=w373) -> ("States Out"=w372:string)  [unwired: 13 in]
        }
        frame "Litho: Order Data" {
          # "Order the Patterns\nUses the ordering data to fix lithography data."
          n168 = control-ref of="Patterns (drag-and-drop reorder)"() -> (w377:refnum<vi>)
          n169 = Unbundle By Name(w380) -> ("Lithography Data"=w378:T8)
          n170 = call "Order Patterns.vi"("error in (no error)"=w376, "Lithography Data"=w378, "ListBox Reference in"=w377) -> ("error out"=w375:errorcluster, "Ordered Lithography Data"=w381:T8)  [unwired: 7 in]
          n171 = Bundle By Name(cluster=w380, "Lithography Data"=w381) -> (w379:T19)
          n172 = call <vilib>:"Add State(s) to Queue__JKI_lib_State_Machine.vi"("State(s) in Front (\"\")"="Driver: Update Controls" ("State(s) in Front (\"\")"), "State(s) in (\"\")"=w383) -> ("States Out"=w382:string)  [unwired: 13 in]
        }
        frame "Litho: Refresh Render" {
          # "Update the images\nUses the lithography data to update the images."
          n173 = Unbundle By Name(w388) -> ("Lithography Data"=w395:T8, "3D.Canvas"=w396:refnum<vi>)
          n174 = control-ref of="Voltage Mapping"() -> (w393:refnum<vi>)
          n175 = local read "Render"() -> (w392:T2)
          n176 = call "Image Generator.vi"("ColorRamp in"=w393, "Lithography Data"=w395, "error in (no error)"=w384, "Image Reference In"=w392) -> ("error out"=w391:errorcluster, "Image Reference Out"=w387:T2)  [unwired: 6 in]
          n177 = local write "Render"(w387) -> ()
          n178 = local read "2D"() -> (w386:T2)
          n179 = call "Convert IMAQ to LV Image.vi"("error in (no error)"=w391, "IMAQImage In (RGB 32)"=w386) -> ("error out"=w389:errorcluster, "Output Image"=w390:T18)  [unwired: 7 in, 1 out]
          n180 = call-poly <vilib>:"Apply Texture.vi"("error in (no error)"=w389, "Image Data"=w390, "Scene Object In"=w396) -> ("error out"=w394:errorcluster)  [unwired: 7 in, 1 out]
          n181 = invoke on="3D Picture" class="SceneGraphDisp (strict)" method="Redraw"(error in=w394) -> (error out=w385:errorcluster)  [unwired: 2 in, 2 out]
          n182 = call <vilib>:"Add State(s) to Queue__JKI_lib_State_Machine.vi"("State(s) in (\"\")"=w398) -> ("States Out"=w397:string)  [unwired: 14 in]
        }
        frame "---------- Driver ----------" {
          # "Template Separator\n(You can make a copy of, or modify, this frame)"
          n183 = call <vilib>:"Add State(s) to Queue__JKI_lib_State_Machine.vi"("State(s) in (\"\")"=w402) -> ("States Out"=w401:string)  [unwired: 14 in]
        }
        frame "Driver: Update Controls" {
          # "Driver is updated to reflect AFM type."
          n184 = Unbundle By Name(w406) -> ("Lithography Data"=w414:T8, "Data Queue"=w413:refnum<queue>)
          n185 = control-ref of="Inkscape File (.svg)"() -> (w412:refnum<vi>)
          n186 = control-ref of="Background Image"() -> (w411:refnum<vi>)
          n187 = property on="AFM Settings" class="SubPnl"() -> ("InsertedVI"=w415:refnum<vi>)  [unwired: 2 in, 2 out]
          n188 = control-ref of="Abort"() -> (w409:refnum<vi>)
          n189 = control-ref of="Run"() -> (w410:refnum<vi>)
          n190 = control-ref of="Run 2"() -> (w403:refnum<vi>)
          n191 = property on="Acquired Data" class="SubPnl"() -> ("InsertedVI"=w404:refnum<vi>)  [unwired: 2 in, 2 out]
          n192 = call "Set Driver Controls.vi"("Background Image"=w411, "Abort"=w409, "Inkscape File (.svg)"=w412, "Run"=w410, "error in (no error)"=w405, "Data Queue"=w413, "Lithography Data"=w414, "VI in"=w415) -> ()  [unwired: 2 in, 2 out]
          n193 = call "Set Driver Controls.vi"("Background Image"=w411, "Abort"=w409, "Inkscape File (.svg)"=w412, "Run"=w403, "Data Queue"=w413, "Lithography Data"=w414, "VI in"=w404) -> ("error out"=w408:errorcluster)  [unwired: 3 in, 1 out]
          n194 = Merge Errors(w408, w405) -> (w407:errorcluster)
          n195 = call <vilib>:"Add State(s) to Queue__JKI_lib_State_Machine.vi"("State(s) in (\"\")"=w417) -> ("States Out"=w416:string)  [unwired: 14 in]
        }
      }
      "Ready?" <- w3
    }
  }
